vi "Start Logger.vi"(8 "error in (no error)":errorcluster, 11 "Worker in":refnum<class "Worker.lvclass">) -> (0 "error out":errorcluster, 2 "File Path":path, 3 "Worker out":refnum<class "Worker.lvclass">)   [LabVIEW 2019, in "Worker.lvclass"]
uses:
  Worker.lvclass
  C:/GitHub/LabActor/Template Module/Template Module.lvclass
  Template Module/Template Module.lvclass/Template Module.ctl
  Worker.lvclass/Worker.ctl
  Loggers/Logger/Logger.lvclass/Logger.ctl
  NHMFL_Core/Libraries/File/File Class/File.lvclass/File.ctl
  Template Module/Read Logger.vi
  Read File prefix.vi
  Read Index digits.vi
  Loggers/Logger/Read File.lvclass.vi
  NHMFL_Core/Libraries/File/File Class/Write File Prefix.vi
  NHMFL_Core/Libraries/File/File Class/Write Index digits.vi
  NHMFL_Core/Libraries/File/File Class/Write Root Data Folder.vi
  Loggers/Logger/Write File.lvclass.vi
  Write File Path.vi
  Template Module/Write Logger.vi
  Read Use buffered logger.vi
  Loggers/Logger/Logger.lvclass
  NHMFL_Core/Libraries/File/File Class/File.lvclass
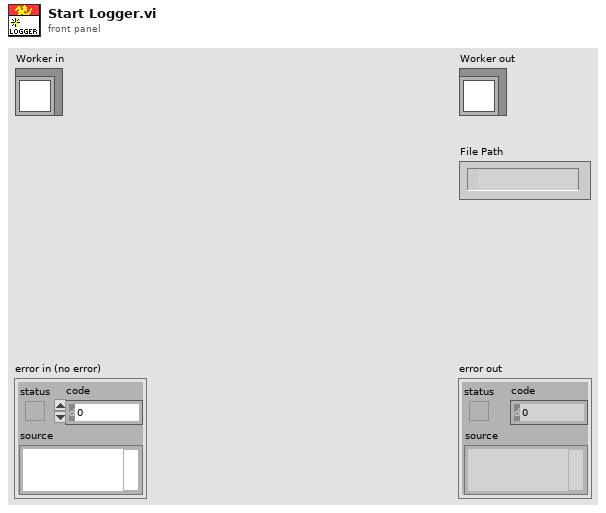
[diagram p1: front panel]
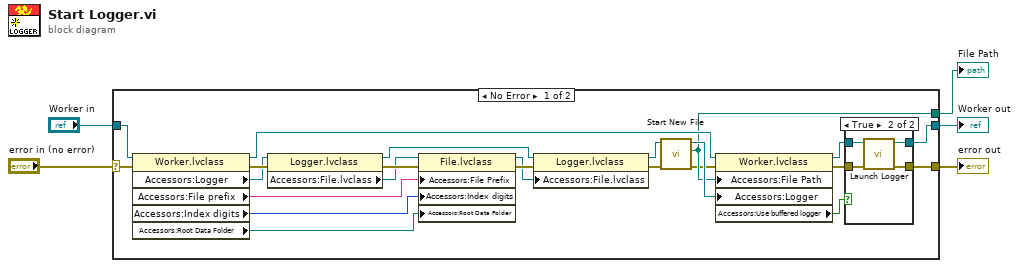
[diagram p0: block diagram]
diagram:
  n1 = case shown="No Error" "error in (no error)" {
    selector: "error in (no error)" -> [w26 w36]
    tunnel: [w9 w36] -> w4
    tunnel: [w8 w35] -> w2
    tunnel: "Worker in" -> [w28 w35]
    tunnel: [w24 _] -> w1
    frame No Error {
      n2 = property class="Worker.lvclass"(reference=w28, error in=w26) -> (reference out=w27:refnum<class "Worker.lvclass">, error out=w23:errorcluster, "Accessors:Logger"=w20:refnum<class "Logger.lvclass">, "Accessors:File prefix"=w13:string, "Accessors:Index digits"=w12:i32, "Accessors:Root Data Folder"=w6:path)
      n3 = property class="Logger.lvclass"(reference=w20, error in=w23) -> (reference out=w18:refnum<class "Logger.lvclass">, error out=w21:errorcluster, "Accessors:File.lvclass"=w15:refnum<class "File.lvclass">)
      n4 = property class="File.lvclass"(reference=w15, error in=w21, "Accessors:File Prefix"=w13, "Accessors:Index digits"=w12, "Accessors:Root Data Folder"=w6) -> (reference out=w14:refnum<class "File.lvclass">, error out=w16:errorcluster)
      n5 = property class="Logger.lvclass"(reference=w18, error in=w16, "Accessors:File.lvclass"=w14) -> (reference out=w17:refnum<class "Logger.lvclass">, error out=w19:errorcluster)
      n6 = call-dynamic "Start New File.vi"("error in (no error)"=w19, "Logger in"=w17) -> ("error out"=w22:errorcluster, "File Path"=w24:path, "Logger out"=w25:refnum<class "Logger.lvclass">)  [unwired: 7 in]
      n7 = property class="Worker.lvclass"(reference=w27, error in=w22, "Accessors:File Path"=w24, "Accessors:Logger"=w25) -> (reference out=w11:refnum<class "Worker.lvclass">, error out=w10:errorcluster, "Accessors:Use buffered logger"=w7:bool)
      n8 = case shown="True" w7 {
        tunnel: w11 -> [w30 w34]
        tunnel: w10 -> [w29 w33]
        tunnel: [w29 w32] -> w9
        tunnel: [w30 w31] -> w8
        frame False {
        }
        frame True {
          n9 = call-dynamic "Launch Logger.vi"("error in (no error)"=w33, "Worker in"=w34) -> ("error out"=w32:errorcluster, "Worker out"=w31:refnum<class "Worker.lvclass">)  [unwired: 8 in]
        }
      }
    }
    frame Error {
    }
  }
  "error out" <- w4
  "Worker out" <- w2
  "File Path" <- w1
